vi "ErrDisplay.vi"(0 "AbortName":string="Abort", 4 "ContName":string="Continue", 5 "eDialogType":T1=enum."Continue", 6 "StopName":string="Stop", 7 "Warning (f)":bool, 8 "Details":string, 9 "Source":string, 10 "Length":i32[](array[numeric]), 11 "Start":i32[](array[numeric])) -> (1 "bStop":bool, 2 "bAbort":bool, 3 "bContinue":bool)   [LabVIEW 2014]
uses:
  <vilib>/Utility/error.llb/ErrWarn.ctl
  eDialogType.ctl
  <vilib>/Utility/miscctls.llb/LVKeyNavTypeDef.ctl
  NISTErrorLib.lvlib
panel:
  in  "btnAbort":bool
  in  "Test for size":string
  in  "truncated & CH message":string="(source truncated; see Context Help window)"
  in  "truncated message":string="(source truncated)"
  in  "description missing (f)":bool
  out "scrollbar text":string
  in  "Stop":bool
  in  "Continue":bool
  out "text":string
  out "Source of Error":string
  out "ErrorOrWarningGlyph":T2
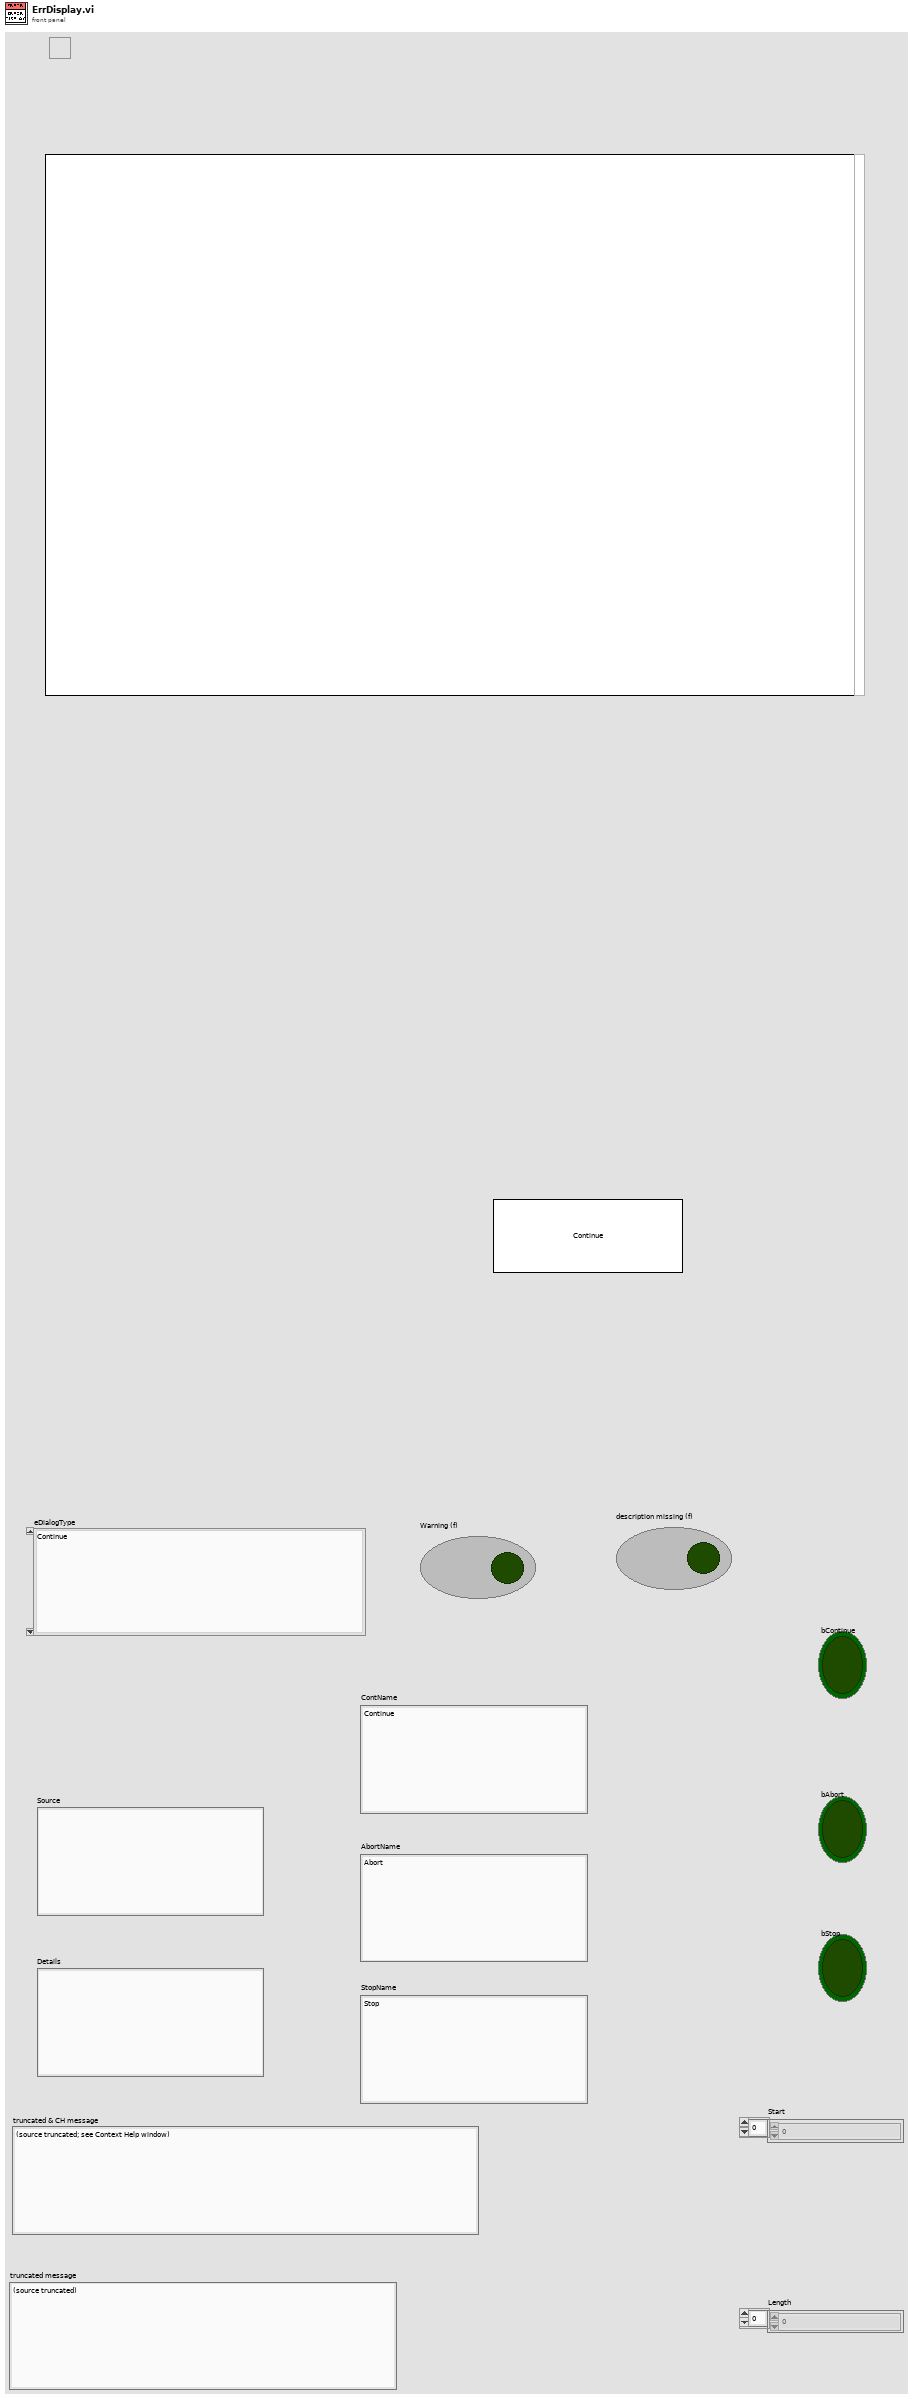
[diagram p1: front panel]
types:
  T1 = typedef "NISTErrorLib.lvlib/eDialogType.ctl" = enum16{"no dialog", "Continue", "Continue,Stop", "Continue,Abort,Stop", "Stop"}
  T2 = typedef "ErrWarn.ctl" = bool
  T3 = typedef "LVKeyNavTypeDef.ctl" = cluster{"Control":bool, "Shift":bool, "Key":string}
  T4 = enum32{"Invalid", "Standard", "Closed", "Hidden", "Minimized", "Maximized"}
  T5 = typedef "LVRectTypeDef.ctl" = cluster{"Left":i16, "Top":i16, "Right":i16, "Bottom":i16}
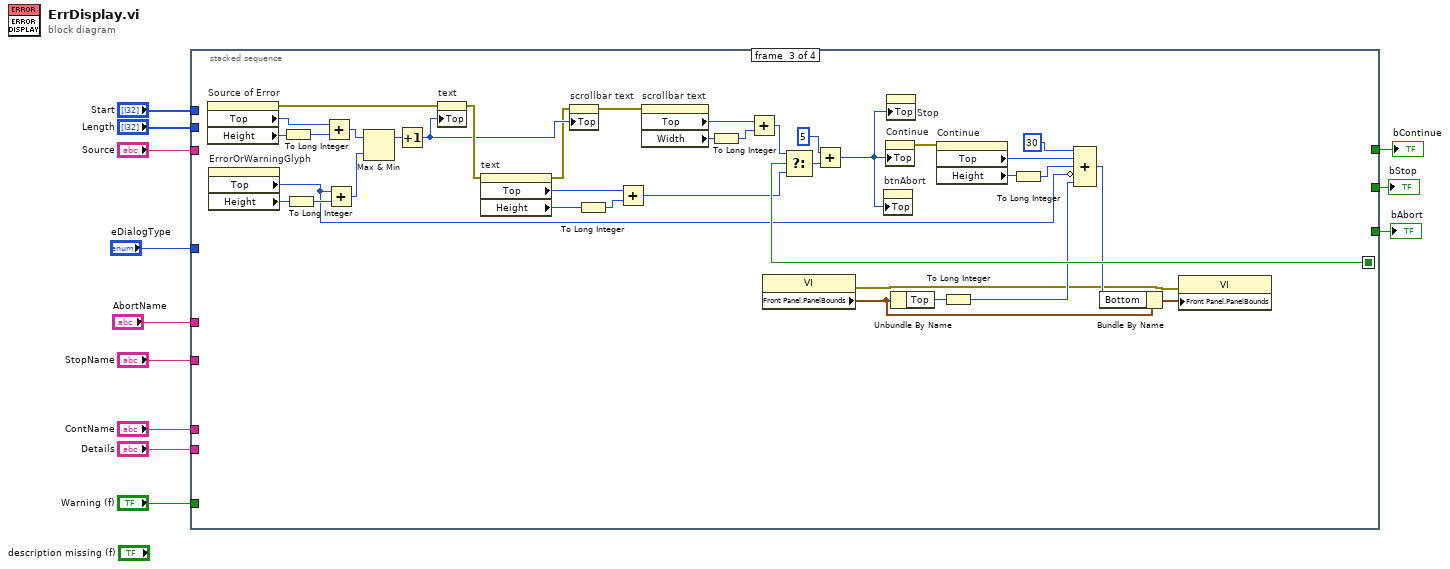
[diagram p0: block diagram]
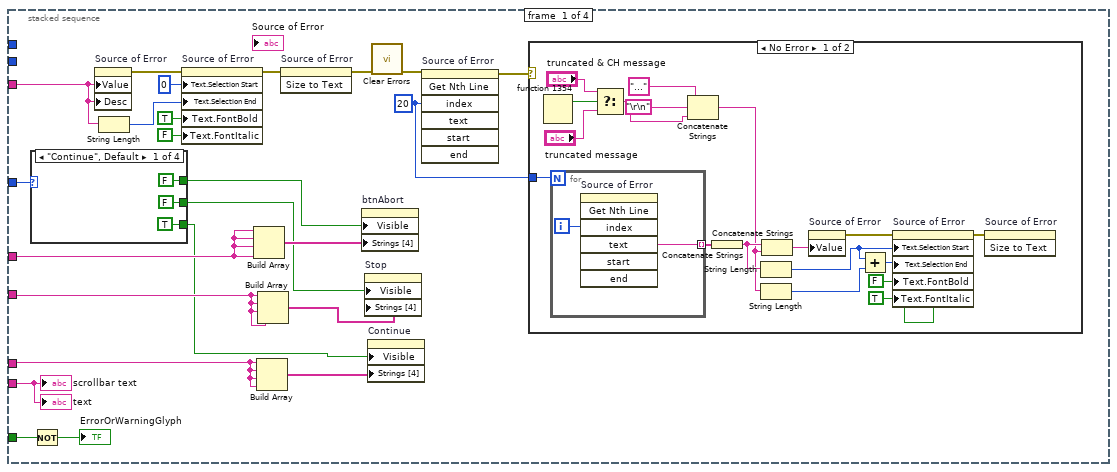
[diagram p2: hidden frame]
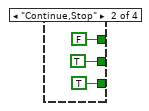
[diagram p3: hidden frame]
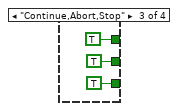
[diagram p4: hidden frame]
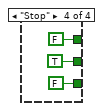
[diagram p5: hidden frame]
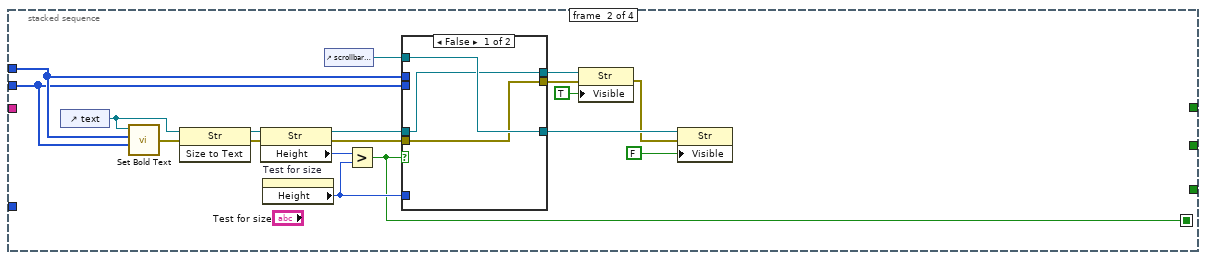
[diagram p7: hidden frame]
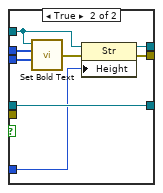
[diagram p8: hidden frame]
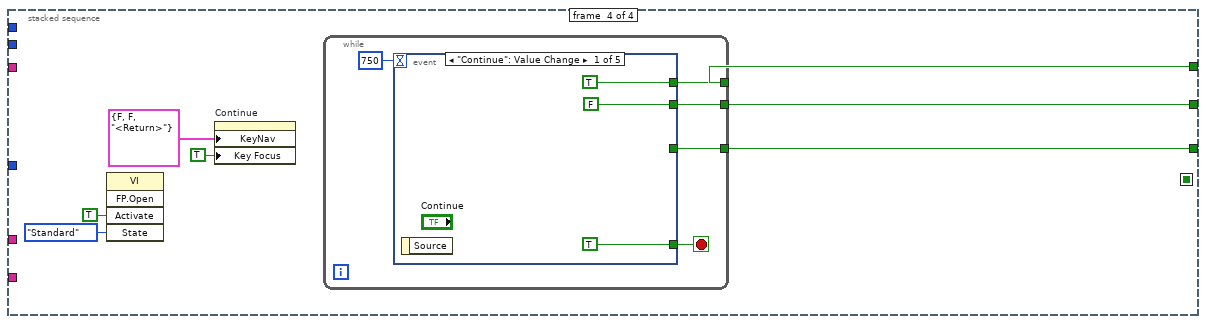
[diagram p9: hidden frame]
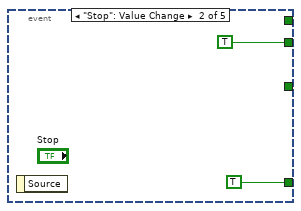
[diagram p10: hidden frame]
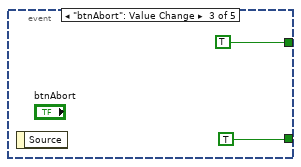
[diagram p11: hidden frame]
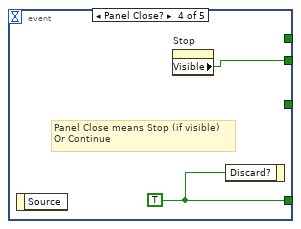
[diagram p12: hidden frame]
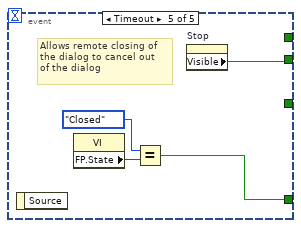
[diagram p13: hidden frame]
diagram:
  n1 = stacked-sequence {
    seq-local: [_ w69 _ _] -> [_ _ w115 _]
    tunnel: "Source" -> [w36 _ _ _]
    tunnel: "Details" -> [w30 _ _ _]
    tunnel: "StopName" -> [w29 _ _ _]
    tunnel: "ContName" -> [w28 _ _ _]
    tunnel: "Start" -> [_ w77 _ _]
    tunnel: "Length" -> [_ w76 _ _]
    tunnel: "Warning (f)" -> [w20 _ _ _]
    tunnel: [_ _ _ w137] -> w5
    tunnel: "eDialogType" -> [w18 _ _ _]
    tunnel: "AbortName" -> [w17 _ _ _]
    tunnel: [_ _ _ w136] -> w2
    tunnel: [_ _ _ w135] -> w1
    frame #0 {
      w21 = u32 20 ("line index")
      n2 = case shown="\"Continue\", Default" w18 {
        tunnel: [TRUE TRUE TRUE FALSE] -> w15
        tunnel: [FALSE TRUE TRUE TRUE] -> w14
        tunnel: [FALSE FALSE TRUE FALSE] -> w13
        frame "Continue", Default {
        }
        frame "Continue,Stop" {
        }
        frame "Continue,Abort,Stop" {
        }
        frame "Stop" {
        }
      }
      n3 = Not(x=w20) -> (.not. x?=→"ErrorOrWarningGlyph":bool)
      n4 = property on="Source of Error" class="Str"("Value"=w36, "Desc"=w36) -> (error out=w33:errorcluster)  [unwired: 2 in, 1 out]
      n5 = String Length(string=w36) -> (length=w31:i32)
      n6 = property on="Source of Error" class="Str"(error in=w33, "Text.Selection Start"=u32 0 ("Text.Selection:Start"), "Text.Selection End"=w31, "Text.FontBold"=TRUE ("Text.Font:Bold"), "Text.FontItalic"=FALSE ("Text.Font:Italic")) -> (error out=w25:errorcluster)  [unwired: 1 in, 1 out]
      n7 = Build Array(w17, w17, w17, w17) -> (w16:string[])
      n8 = Build Array(w28, w28, w28, w28) -> (w26:string[])
      n9 = Build Array(w29, w29, w29, w29) -> (w27:string[])
      n10 = invoke on="Source of Error" class="Str" method="Size to Text"(error in=w25) -> (error out=w24:errorcluster)  [unwired: 2 in, 2 out]
      n11 = property on="btnAbort" class="Bool"("Visible"=w13, "Strings [4]"=w16) -> ()  [unwired: 2 in, 2 out]
      n12 = property on="Stop" class="Bool"("Visible"=w14, "Strings [4]"=w27) -> ()  [unwired: 2 in, 2 out]
      n13 = property on="Continue" class="Bool"("Visible"=w15, "Strings [4]"=w26) -> ()  [unwired: 2 in, 2 out]
      n14 = call <vilib>:"Clear Errors.vi"("error in (no error)"=w24) -> ("error out"=w23:errorcluster)  [unwired: 5 in, 1 out]
      n15 = invoke on="Source of Error" class="Str" method="Get Nth Line"(error in=w23, "index"=w21) -> (error out=w22:errorcluster)  [unwired: 5 in, 6 out]
      n16 = case shown="No Error" w22 {
        tunnel: w21 -> [w60 _]
        frame No Error {
          n17 = fn#1354() -> (1:w66:bool)  [unwired: 1 out]
          n18 = for {
            N: w60 -> [_]
            tunnel: [w67] -> w59 mode=indexing
            i -> [w68]
            n19 = invoke on="Source of Error" class="Str" method="Get Nth Line"("index"=w68) -> ("text"=w67:string)  [unwired: 6 in, 6 out]
          }
          n20 = Select(t="truncated & CH message", s=w66, f="truncated message") -> (s? t:f=w61:string)
          n21 = Concatenate Strings("..." ("string"), "\r\n", w61) -> (w57:string)
          n22 = Concatenate Strings(w59) -> (w58:string)
          n23 = String Length(string=w58) -> (length=w53:i32)
          n24 = String Length(string=w57) -> (length=w52:i32)
          n25 = Concatenate Strings(w58, w57) -> (w56:string)
          n26 = property on="Source of Error" class="Str"("Value"=w56) -> (error out=w55:errorcluster)  [unwired: 2 in, 1 out]
          n27 = Add(x=w53, y=w52) -> (x+y=w54:i32)
          n28 = property on="Source of Error" class="Str"(error in=w55, "Text.Selection Start"=w53, "Text.Selection End"=w54, "Text.FontBold"=FALSE ("Text.Font:Bold"), "Text.FontItalic"=TRUE ("Text.Font:Italic")) -> (error out=w49:errorcluster)  [unwired: 1 in, 1 out]
          n29 = invoke on="Source of Error" class="Str" method="Size to Text"(error in=w49) -> ()  [unwired: 2 in, 3 out]
        }
        frame Error {
        }
      }
      "scrollbar text" <- w30
      "text" <- w30
    }
    frame #1 {
      n30 = control-ref of="text"() -> (w86:refnum<vi>)
      n31 = call <vilib>:"Set Bold Text.vi"("Length"=w76, "Start"=w77, "text"=w86) -> ("error out"=w85:errorcluster)  [unwired: 3 in]
      n32 = invoke class="Str" method="Size to Text"(reference=w86, error in=w85) -> (reference out=w84:refnum<vi>, error out=w83:errorcluster)  [unwired: 1 in, 1 out]
      n33 = property class="Str"(reference=w84, error in=w83) -> (reference out=w80:refnum<vi>, error out=w81:errorcluster, "Height"=w82:u32)
      n34 = property on="Test for size" class="Str"() -> ("Height"=w79:u32)  [unwired: 2 in, 2 out]
      n35 = control-ref of="scrollbar text"() -> (w78:refnum<vi>)
      n36 = Greater?(x=w82, y=w79) -> (0:w69:bool)
      n37 = case shown="False" w69 {
        tunnel: w81 -> [w87 _]
        tunnel: w80 -> [w88 w91]
        tunnel: w79 -> [_ w90]
        tunnel: w78 -> [w89 w94]
        tunnel: w77 -> [_ w97]
        tunnel: w76 -> [_ w96]
        tunnel: [w88 w93] -> w75
        tunnel: [w87 w92] -> w74
        tunnel: [w89 w91] -> w72
        frame False {
        }
        frame True {
          n38 = call <vilib>:"Set Bold Text.vi"("Length"=w96, "Start"=w97, "text"=w94) -> ("error out"=w95:errorcluster)  [unwired: 3 in]
          n39 = property class="Str"(reference=w94, error in=w95, "Height"=w90) -> (reference out=w93:refnum<vi>, error out=w92:errorcluster)
        }
      }
      n40 = property class="Str"(reference=w75, error in=w74, "Visible"=TRUE) -> (error out=w71:errorcluster)  [unwired: 1 out]
      n41 = property class="Str"(reference=w72, error in=w71, "Visible"=FALSE) -> ()  [unwired: 2 out]
    }
    frame #2 {
      n42 = property on="Source of Error" class="Str"() -> (error out=w126:errorcluster, "Top"=w131:i32, "Height"=w134:u32)  [unwired: 2 in, 1 out]
      n43 = property on="ErrorOrWarningGlyph" class="Bool"() -> ("Top"=w105:i32, "Height"=w133:u32)  [unwired: 2 in, 2 out]
      n44 = To Long Integer(number=w134) -> (32bit integer=w132:i32)
      n45 = To Long Integer(number=w133) -> (32bit integer=w130:i32)
      n46 = Add(x=w131, y=w132) -> (x+y=w129:i32)
      n47 = Add(x=w105, y=w130) -> (x+y=w128:i32)
      n48 = Max & Min(x=w129, y=w128) -> (max(x,y)=w127:i32)  [unwired: 1 out]
      n49 = Increment(x=w127) -> (x+1=w124:i32)
      n50 = property on="text" class="Str"(error in=w126, "Top"=w124) -> (error out=w125:errorcluster)  [unwired: 1 in, 1 out]
      n51 = property on="text" class="Str"(error in=w125) -> (error out=w123:errorcluster, "Top"=w117:i32, "Height"=w121:u32)  [unwired: 1 in, 1 out]
      n52 = property on="scrollbar text" class="Str"(error in=w123, "Top"=w124) -> (error out=w122:errorcluster)  [unwired: 1 in, 1 out]
      n53 = To Long Integer(number=w121) -> (32bit integer=w119:i32)
      n54 = Add(x=w117, y=w119) -> (x+y=w113:i32)
      n55 = property on="scrollbar text" class="Str"(error in=w122) -> ("Top"=w116:i32, "Width"=w120:u32)  [unwired: 1 in, 2 out]
      n56 = To Long Integer(number=w120) -> (32bit integer=w118:i32)
      n57 = Add(x=w116, y=w118) -> (x+y=w114:i32)
      n58 = property class="VI"() -> (error out=w99:errorcluster, "Front Panel.PanelBounds"=w101:T5)  [unwired: 2 in, 1 out]
      n59 = Select(t=w114, s=w115, f=w113) -> (s? t:f=w112:i32)
      n60 = Add(x=5, y=w112) -> (x+y=w98:i32)
      n61 = property on="btnAbort" class="Bool"("Top"=w98) -> ()  [unwired: 2 in, 2 out]
      n62 = property on="Continue" class="Bool"("Top"=w98) -> (error out=w110:errorcluster)  [unwired: 2 in, 1 out]
      n63 = property on="Stop" class="Bool"("Top"=w98) -> ()  [unwired: 2 in, 2 out]
      n64 = Unbundle By Name(w101) -> ("Top"=w104:i16)
      n65 = property on="Continue" class="Bool"(error in=w110) -> ("Top"=w107:i32, "Height"=w109:u32)  [unwired: 1 in, 2 out]
      n66 = To Long Integer(number=w104) -> (32bit integer=w103:i32)
      n67 = To Long Integer(number=w109) -> (32bit integer=w108:i32)
      n68 = Compound Arithmetic op=ADD(30 ("value"), w107, w108, invert w105, w103) -> (w102:i32)
      n69 = Bundle By Name(cluster=w101, "Bottom"=w102) -> (w100:T5)
      n70 = property class="VI"(error in=w99, "Front Panel.PanelBounds"=w100) -> ()  [unwired: 1 in, 2 out]
    }
    frame #3 {
      n71 = invoke class="VI" method="FP.Open"("Activate"=TRUE ("Activate?"), "State"=T4."Standard") -> ()  [unwired: 3 in, 5 out]
      n72 = property on="Continue" class="Bool"("KeyNav"=T3 {"Control"=FALSE, "Shift"=FALSE, "Key"="<Return>"} ("Focus Key Binding"), "Key Focus"=TRUE) -> ()  [unwired: 2 in, 2 out]
      n73 = while {
        tunnel: [w145] -> w137
        tunnel: [w143] -> w136
        tunnel: [w142] -> w135
        stop <- w146 stop-if-true
        n74 = event shown="[0] \"Continue\": Value Change" {
          selector: _ -> [_ _ _ _ _]
          dyn-events: _ -> [_ _ _ _ _]
          timeout: 750 -> [_ _ _ _ _]
          tunnel: [TRUE TRUE TRUE w154 w157] -> w146
          tunnel: [FALSE TRUE _ w155 w156] -> w145
          tunnel: [TRUE _ _ _ _] -> w143
          tunnel: [_ _ TRUE _ _] -> w142
          event "Continue": Value Change {
            n75 = event-data() -> ()  [unwired: 1 in, 1 out]
          }
          event "Stop": Value Change {
            n76 = event-data() -> ()  [unwired: 1 in, 1 out]
          }
          event "btnAbort": Value Change {
            n77 = event-data() -> ()  [unwired: 1 in, 1 out]
          }
          event Panel Close? {
            w154 = TRUE
            # "Panel Close means Stop (if visible)\nOr Continue"
            n78 = event-data() -> ()  [unwired: 1 in, 1 out]
            n79 = property on="Stop" class="Bool"() -> ("Visible"=w155:bool)  [unwired: 2 in, 2 out]
            n80 = event-data("Discard?"=w154) -> ()  [unwired: 1 in, 1 out]
          }
          event Timeout {
            # "Allows remote closing of\nthe dialog to cancel out \nof the dialog"
            n81 = event-data() -> ()  [unwired: 1 in, 1 out]
            n82 = property class="VI"() -> ("FP.State"=w159:T4)  [unwired: 2 in, 2 out]
            n83 = Equal?(x=T4."Closed" ("Front Panel Window:State"), y=w159) -> (x = y?=w157:bool)
            n84 = property on="Stop" class="Bool"() -> ("Visible"=w156:bool)  [unwired: 2 in, 2 out]
          }
        }
      }
    }
  }
  "bStop" <- w5
  "bAbort" <- w1
  "bContinue" <- w2
